vi "ADC10 LaunchPad.vi"(11 "string":string) -> (2 "ADC10 (Volt)":dbl, 3 "ADCvalue":u16)   [LabVIEW 2010]
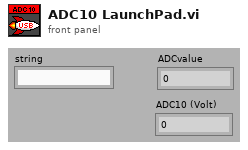
[diagram p1: front panel]
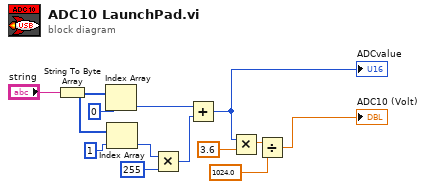
[diagram p0: block diagram]
diagram:
  n1 = String To Byte Array(string="string") -> (unsigned byte array=w12:u8[])
  n2 = Index Array(array=w12, index=0) -> (element=w7:u8)
  n3 = Index Array(array=w12, index=1) -> (element=w10:u8)
  n4 = Multiply(x=w10, y=u16 255) -> (x*y=w8:u16)
  n5 = Add(x=w7, y=w8) -> (x+y=w6:u16)
  "ADCvalue" <- w6
  n6 = Multiply(x=w6, y=3.6) -> (x*y=w4:dbl)
  n7 = Divide(x=w4, y=1024.0) -> (x/y=→"ADC10 (Volt)":dbl)
